vi "imaqrio_OpenImpl.vi"(1 "VI in Hardware":path=path "fpgaadd.vi", 2 "VI Signature Created For":u8[](array[numeric]), 4 "HW Exec Input":refnum<visa-resource-name>, 5 "Warnings Wanted (T)":bool=TRUE, 6 "error in (no error)":errorcluster, 7 "7100 Device Index (0)":i32, 8 "Open Options (Open, Download, Run)":T1(ring)=enum."Open, Download, Run", 9 "Exec Options (Hardware)":enum16{"Hardware", "Simulation"}(ring), 10 "use external input":bool) -> (0 "error out":errorcluster, 3 "HW Exec Ref Out":refnum<visa-resource-name>)   [LabVIEW 2017]
doc: "This VI Opens a reference to the \"VI in Hardware\" that can either be run in hardware or software. Use the software option to simulate your system design.\nIf you don't want a dialog to pop up when the VI for hardware has changed since you last ran the host interface utility set the \"warnings wanted\" parameter to False.\nAs long as you are on the same machine, this sub VI can be run just using the default parameter values. The default value for the \"VI in Hardware\" path is the absolute path to the VI you specified when you ran the host interface utility. If your VI will be run on a different machine, you should make this path relative. The default open options are: Open, Download, and then Run."
panel:
  # "In Simulation the Hardware VI just gets run in the host LabVIEW execution\nenvironment."
  # "Setting to true will create a warning dialog if the vi signatures don't\nmatch between the hardware VI and the hardware VI this was originally\ncreated for."
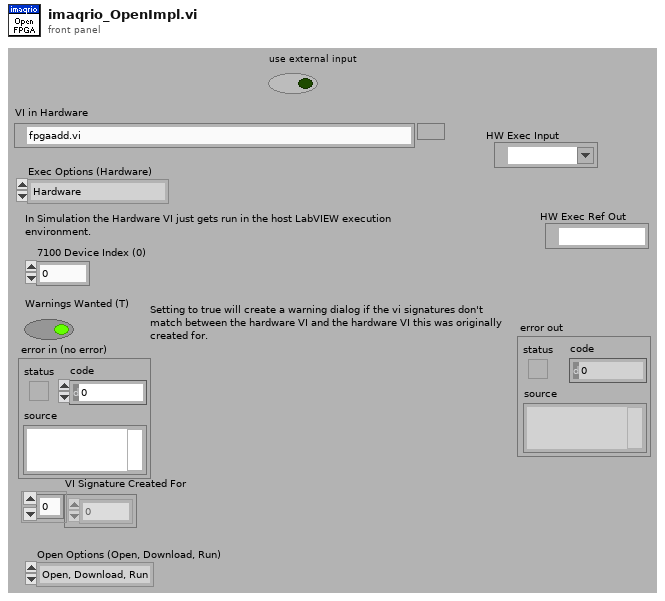
[diagram p1: front panel]
types:
  T1 = enum16{"Open", "Open, Download", "Open, Download, Run"}
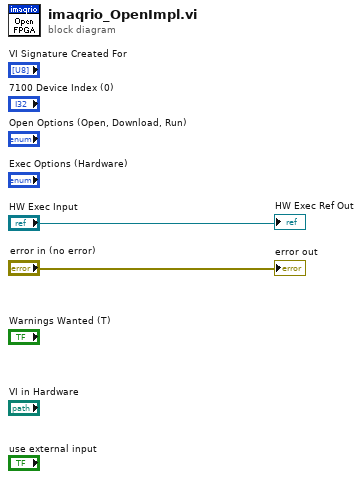
[diagram p0: block diagram]
diagram:
  "error out" <- "error in (no error)"
  "HW Exec Ref Out" <- "HW Exec Input"
